vi "CC Rd Wr Observation List.vi"(8 "error in (no error)":errorcluster, 9 "filepath":path, 10 "Write? (F:Read)":bool, 11 "Observation List":T1[](array[typedef])) -> (0 "error out":errorcluster, 1 "file":path, 2 "Errors":string[](array[string]), 3 "Observation List":T1[](array[typedef]))   [LabVIEW 2021]
uses:
  typedefs/CC cluster Observation.ctl
  Observation Queue/CC enum Observation Status.ctl
  Telescope/CC cluster Telescope Offsets.ctl
  typedefs/CC cluster Observation Dither Options.ctl
  typedefs/CC enum Dither Selection.ctl
  <vilib>/Utility/file.llb/Write Delimited Spreadsheet (string).vi
panel:
  out "Header":string[](array[string])
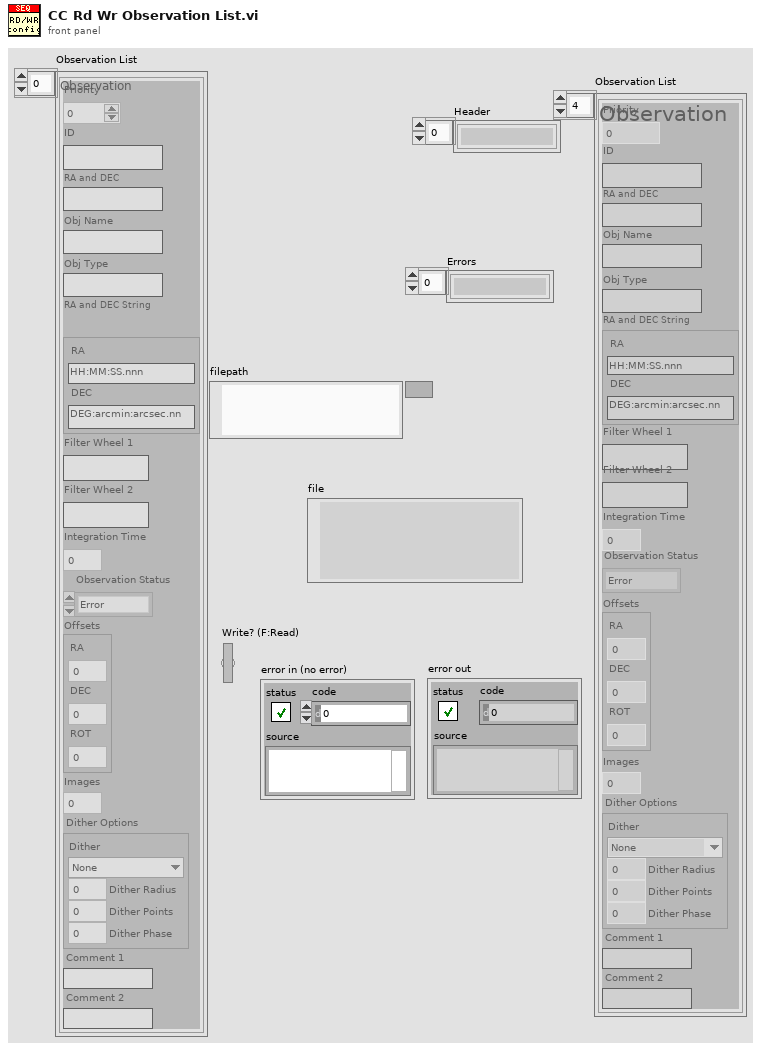
[diagram p1: front panel]
types:
  T1 = typedef "CC cluster Observation.ctl" = cluster{"Priority":i32, "ID":string, "Observer":string, "Obj Name":string, "Obj Type":string, "RA and DEC String":cluster{"RA":string, "DEC":string}, "Filter Wheel 1":string, "Filter Wheel 2":string, "Integration Time":dbl, "Observation Status":T2, "Offsets":T3, "Images":i32, "Dither Options":T4, "Comment 1":string, "Comment 2":string}
  T2 = typedef "CC enum Observation Status.ctl" = enum16{"Ready", "Running", "Done", "Error"}
  T3 = typedef "CC cluster Telescope Offsets.ctl" = cluster{"RA":dbl, "DEC":dbl, "ROT":dbl}
  T4 = typedef "CC cluster Observation Dither Options.ctl" = cluster{"Dither":T5, "Dither Radius":dbl, "Dither Points":i32, "Dither Phase":dbl}
  T5 = typedef "CC enum Dither Selection.ctl" = enum16{"None", "Circle", "Random"}
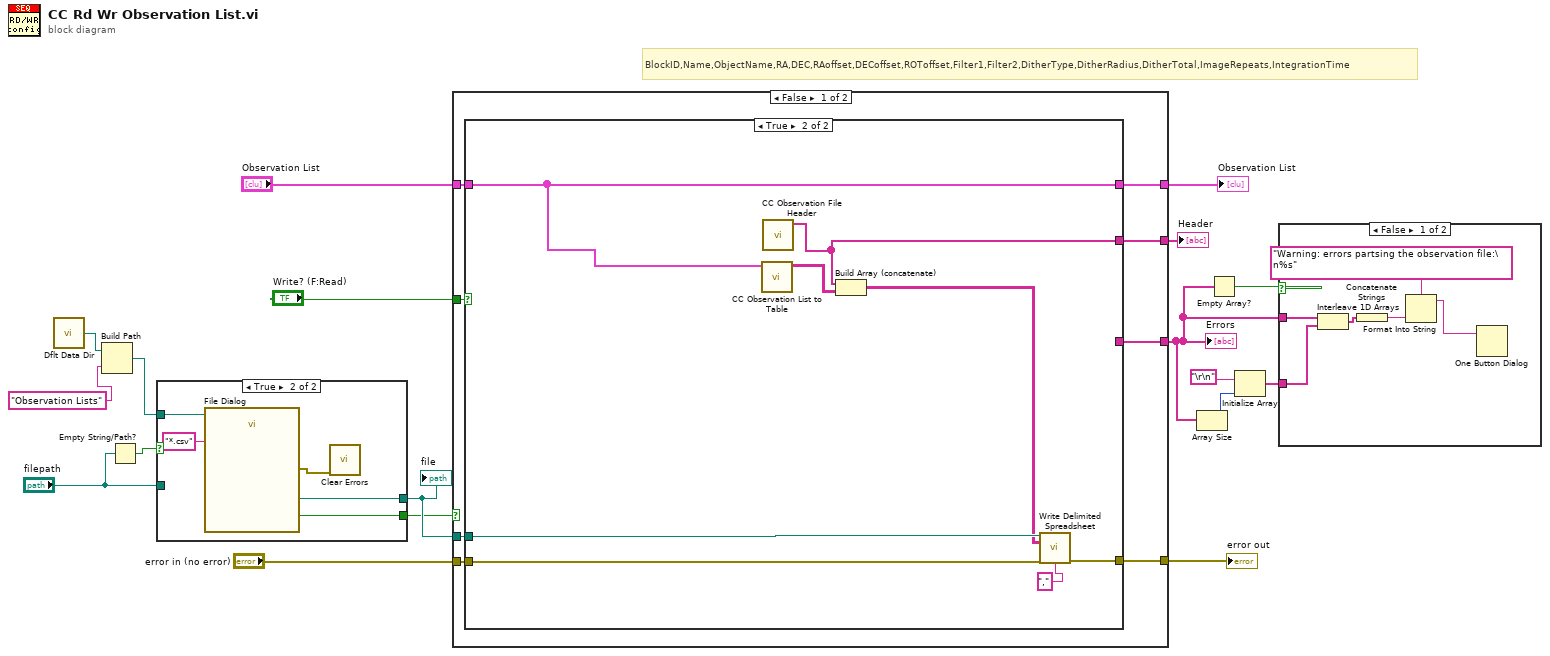
[diagram p0: block diagram]
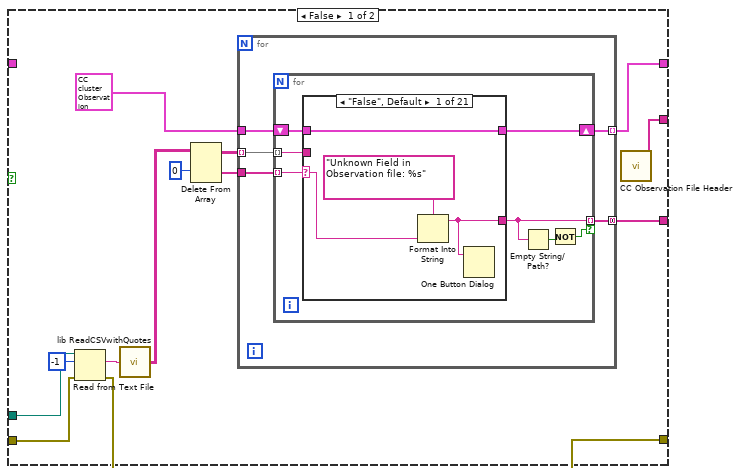
[diagram p3: hidden frame]
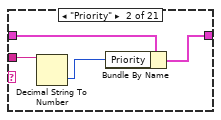
[diagram p4: hidden frame]
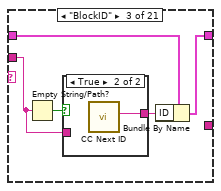
[diagram p5: hidden frame]
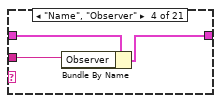
[diagram p7: hidden frame]
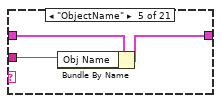
[diagram p8: hidden frame]
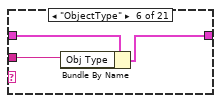
[diagram p9: hidden frame]
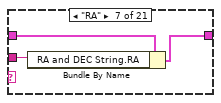
[diagram p10: hidden frame]
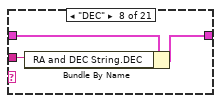
[diagram p11: hidden frame]
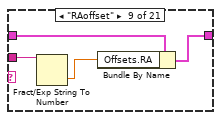
[diagram p12: hidden frame]
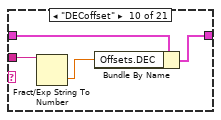
[diagram p13: hidden frame]
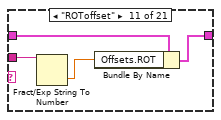
[diagram p14: hidden frame]
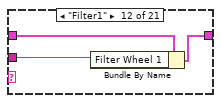
[diagram p15: hidden frame]
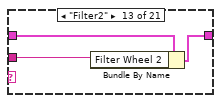
[diagram p16: hidden frame]
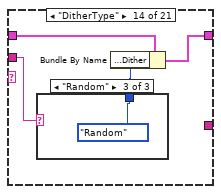
[diagram p17: hidden frame]
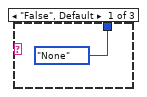
[diagram p18: hidden frame]
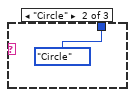
[diagram p19: hidden frame]
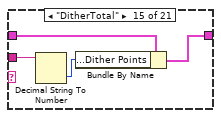
[diagram p20: hidden frame]
diagram:
  # "BlockID,Name,ObjectName,RA,DEC,RAoffset,DECoffset,ROToffset,Filter1,Filter2,DitherType,DitherRadius,DitherTotal,ImageRepeats,IntegrationTime"
  n1 = call <vilib>:"Dflt Data Dir.vi"() -> ("App:Default Data Directory"=w10:path)
  n2 = Build Path(base path=w10, name or relative path="Observation Lists") -> (appended path=w8:path)
  n3 = Empty String/Path?(string/path="filepath") -> (empty?=w13:bool)
  n4 = case shown="True" w13 {
    tunnel: [w19 w24] -> w12
    tunnel: "filepath" -> [w19 _]
    tunnel: w8 -> [_ w23]
    tunnel: [_ w21] -> w7
    frame False {
    }
    frame True {
      n5 = call "File Dialog"("start path"=w23, "pattern (all files)"="*.csv") -> ("selected path"=w24:path, "cancelled"=w21:bool, "error out"=w20:errorcluster)  [unwired: 10 in, 1 out]
      n6 = call <vilib>:"Clear Errors.vi"("error in (no error)"=w20) -> ()  [unwired: 5 in, 2 out]
    }
  }
  "file" <- w12
  n7 = case shown="False" w7 {
    tunnel: "error in (no error)" -> [w32 w147]
    tunnel: "Write? (F:Read)" -> [w31 _]
    tunnel: "Observation List" -> [w30 w148]
    tunnel: [w29 w147] -> w15
    tunnel: [w28 w148] -> w14
    tunnel: w12 -> [w27 _]
    tunnel: [w26 _] -> w3
    tunnel: [w25 _] -> w6
    frame False {
      n8 = case shown="True" w31 {
        tunnel: w32 -> [w33 w146]
        tunnel: w30 -> [_ w142]
        tunnel: w27 -> [w38 w145]
        tunnel: [w34 w144] -> w29
        tunnel: [w41 w142] -> w28
        tunnel: [w40 _] -> w26
        tunnel: [w39 w140] -> w25
        frame False {
          n9 = Read from Text File(file (use dialog)=w38, count=-1, error in=w33) -> (text=w37:string, error out=w34:errorcluster)  [unwired: 1 in, 2 out]
          n10 = call "lib ReadCSVwithQuotes.vi"("String"=w37) -> ("Array"=w35:string[][])  [unwired: 4 in]
          n11 = Delete From Array(array=w35, index (row)=0) -> (deleted portion=w43:string[], array with subset deleted=w42:string[][])  [unwired: 2 in]
          n12 = for {
            tunnel: T1 {"Priority"=0, "ID"="", "Observer"="", "Obj Name"="", "Obj Type"="", "RA and DEC String"={"RA"="12:34:56.789", "DEC"="010:11:12.013"}, "Filter Wheel 1"="", "Filter Wheel 2"="", "Integration Time"=0.0, "Observation Status"=enum."Ready", "Offsets"={"RA"=0.0, "DEC"=0.0, "ROT"=0.0}, "Images"=0, "Dither Options"={"Dither"=enum."Random", "Dither Radius"=0.0, "Dither Points"=0, "Dither Phase"=0.0}, "Comment 1"="", "Comment 2"=""} ("Observation") -> [w50]
            tunnel: w43 -> [w49]
            tunnel: w42 -> [w48] mode=indexing
            tunnel: [w47] -> w41 mode=indexing
            tunnel: [w46] -> w40 mode=concatenating
            n13 = for {
              shift-right: [w54] -> w47
              shift-left: w50 -> [w55]
              tunnel: w49 -> [w57] mode=indexing
              tunnel: w48 -> [w56] mode=indexing
              tunnel: [w53] -> w46 mode=indexing if=w51
              n14 = case shown="\"False\", Default" w57 {
                selector: w57 -> [w60 _ _ _ _ _ _ _ _ _ _ _ _ _ _ _ _ _ _ _ _]
                tunnel: w56 -> [_ w63 w66 w73 w76 w79 w82 w85 w89 w93 w97 w100 w103 w106 w114 w118 w122 w126 w130 w134 w137]
                tunnel: w55 -> [w59 w65 w70 w75 w78 w81 w84 w87 w91 w95 w99 w102 w105 w109 w116 w120 w124 w128 w132 w135 w138]
                tunnel: [w59 w64 w69 w74 w77 w80 w83 w86 w90 w94 w98 w101 w104 w108 w115 w119 w123 w127 w131 w133 w136] -> w54
                tunnel: [w58 _ _ _ _ _ _ _ _ _ _ _ _ _ _ _ _ _ _ _ _] -> w53
                frame "False", Default {
                  n15 = Format Into String(format string="Unknown Field in Observation file: %s", w60) -> (resulting string=w58:string)  [unwired: 2 in, 1 out]
                  n16 = One Button Dialog(message=w58) -> ()  [unwired: 1 in, 1 out]
                }
                frame "Priority" {
                  n17 = Decimal String To Number(string=w63) -> (number=w62:i32)  [unwired: 2 in, 1 out]
                  n18 = Bundle By Name(cluster=w65, "Priority"=w62) -> (w64:T1)
                }
                frame "BlockID" {
                  n19 = Empty String/Path?(string/path=w66) -> (empty?=w68:bool)
                  n20 = case shown="True" w68 {
                    tunnel: [w71 w72] -> w67
                    tunnel: w66 -> [w71 _]
                    frame False {
                    }
                    frame True {
                      n21 = call "CC Next ID.vi"() -> ("BlockID string"=w72:string)  [unwired: 9 in, 2 out]
                    }
                  }
                  n22 = Bundle By Name(cluster=w70, "ID"=w67) -> (w69:T1)
                }
                frame "Name", "Observer" {
                  n23 = Bundle By Name(cluster=w75, "Observer"=w73) -> (w74:T1)
                }
                frame "ObjectName" {
                  n24 = Bundle By Name(cluster=w78, "Obj Name"=w76) -> (w77:T1)
                }
                frame "ObjectType" {
                  n25 = Bundle By Name(cluster=w81, "Obj Type"=w79) -> (w80:T1)
                }
                frame "RA" {
                  n26 = Bundle By Name(cluster=w84, "RA and DEC String.RA"=w82) -> (w83:T1)
                }
                frame "DEC" {
                  n27 = Bundle By Name(cluster=w87, "RA and DEC String.DEC"=w85) -> (w86:T1)
                }
                frame "RAoffset" {
                  n28 = Fract/Exp String To Number(string=w89) -> (number=w88:dbl)  [unwired: 3 in, 1 out]
                  n29 = Bundle By Name(cluster=w91, "Offsets.RA"=w88) -> (w90:T1)
                }
                frame "DECoffset" {
                  n30 = Fract/Exp String To Number(string=w93) -> (number=w92:dbl)  [unwired: 3 in, 1 out]
                  n31 = Bundle By Name(cluster=w95, "Offsets.DEC"=w92) -> (w94:T1)
                }
                frame "ROToffset" {
                  n32 = Fract/Exp String To Number(string=w97) -> (number=w96:dbl)  [unwired: 3 in, 1 out]
                  n33 = Bundle By Name(cluster=w99, "Offsets.ROT"=w96) -> (w98:T1)
                }
                frame "Filter1" {
                  n34 = Bundle By Name(cluster=w102, "Filter Wheel 1"=w100) -> (w101:T1)
                }
                frame "Filter2" {
                  n35 = Bundle By Name(cluster=w105, "Filter Wheel 2"=w103) -> (w104:T1)
                }
                frame "DitherType" {
                  n36 = case shown="\"Random\"" w106 {
                    tunnel: [enum16{"None", "Circle", "Random"}."None" ("Dither Options.Type") enum16{"None", "Circle", "Random"}."Circle" ("Dither Options.Type") enum16{"None", "Circle", "Random"}."Random" ("Dither Options.Type")] -> w107
                    frame "False", Default {
                    }
                    frame "Circle" {
                    }
                    frame "Random" {
                    }
                  }
                  n37 = Bundle By Name(cluster=w109, "Dither Options.Dither"=w107) -> (w108:T1)
                }
                frame "DitherTotal" {
                  n38 = Decimal String To Number(string=w114) -> (number=w113:i32)  [unwired: 2 in, 1 out]
                  n39 = Bundle By Name(cluster=w116, "Dither Options.Dither Points"=w113) -> (w115:T1)
                }
                frame "DitherRadius" {
                  n40 = Fract/Exp String To Number(string=w118) -> (number=w117:dbl)  [unwired: 3 in, 1 out]
                  n41 = Bundle By Name(cluster=w120, "Dither Options.Dither Radius"=w117) -> (w119:T1)
                }
                frame "DitherPhase" {
                  n42 = Fract/Exp String To Number(string=w122) -> (number=w121:dbl)  [unwired: 3 in, 1 out]
                  n43 = Bundle By Name(cluster=w124, "Dither Options.Dither Phase"=w121) -> (w123:T1)
                }
                frame "Images" {
                  n44 = Decimal String To Number(string=w126) -> (number=w125:i32)  [unwired: 2 in, 1 out]
                  n45 = Bundle By Name(cluster=w128, "Images"=w125) -> (w127:T1)
                }
                frame "IntegrationTime" {
                  n46 = Fract/Exp String To Number(string=w130) -> (number=w129:dbl)  [unwired: 3 in, 1 out]
                  n47 = Bundle By Name(cluster=w132, "Integration Time"=w129) -> (w131:T1)
                }
                frame "Comment1" {
                  n48 = Bundle By Name(cluster=w135, "Comment 1"=w134) -> (w133:T1)
                }
                frame "Comment2" {
                  n49 = Bundle By Name(cluster=w138, "Comment 1"=w137) -> (w136:T1)
                }
              }
              n50 = Empty String/Path?(string/path=w53) -> (empty?=w52:bool)
              n51 = Not(x=w52) -> (.not. x?=w51:bool)
            }
          }
          n52 = call "CC Observation File Header.vi"() -> ("Header"=w39:string[])  [unwired: 10 in, 1 out]
        }
        frame True {
          n53 = call "CC Observation List to Table.vi"("Observation List"=w142) -> ("File Ready Table"=w139:string[][])  [unwired: 7 in, 3 out]
          n54 = call "CC Observation File Header.vi"() -> ("Header"=w140:string[])  [unwired: 10 in, 1 out]
          n55 = Build Array (concatenate)(w140, w139) -> (w141:string[][])
          n56 = call-poly <vilib>:"Write Delimited Spreadsheet.vi"("file path (dialog if empty)"=w145, "2D data"=w141, "error in (no error)"=w146, "delimiter (\\t)"="," ("delimiter (\\t)")) -> ("error out"=w144:errorcluster)  [unwired: 10 in, 1 out]
        }
      }
    }
    frame True {
    }
  }
  "error out" <- w15
  "Observation List" <- w14
  "Errors" <- w3
  "Header" <- w6
  n57 = Array Size(array=w3) -> (size(s)=w2:i32)
  n58 = Empty Array?(array=w3) -> (empty?=w5:bool)
  n59 = Initialize Array("\r\n", w2) -> (w1:string[])
  n60 = case shown="False" w5 {
    tunnel: w3 -> [w154 _]
    tunnel: w1 -> [w153 _]
    frame False {
      n61 = Interleave 1D Arrays(w154, w153) -> (w151:string[])
      n62 = Concatenate Strings(w151) -> (w150:string)
      n63 = Format Into String(format string="Warning: errors partsing the observation file:\n%s", w150) -> (resulting string=w149:string)  [unwired: 2 in, 1 out]
      n64 = One Button Dialog(message=w149) -> ()  [unwired: 1 in, 1 out]
    }
    frame True {
    }
  }
